vi "Turret_Globals.vi"() -> ()   [LabVIEW 2019]
uses:
  Subsystems/Turret/Turret_Cluster.ctl
panel:
  in  "Turret_Execute_Notifier":refnum<notifier>
  in  "Turret_Set_Notifier":refnum<notifier>
  in  "Turret_Execute_Ref":string="Turret_Execute_Ref"
  in  "Turret_Set_Ref":string
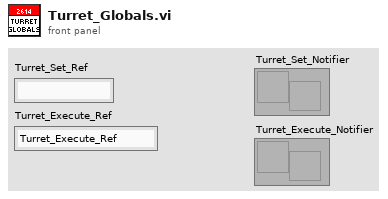
[diagram p1: front panel]
diagram:
